vi "DP-Plot I-O.vi"(0 "Input Array (4xn)":dbl[][](array[numeric]) format="%.2f") -> (1 "Current I-O Plot":cluster{cluster{dbl, dbl}[]}[](graph), 2 "All-freq I-O Plot":cluster{cluster{dbl, dbl}[]}[](graph))   [LabVIEW 2020]
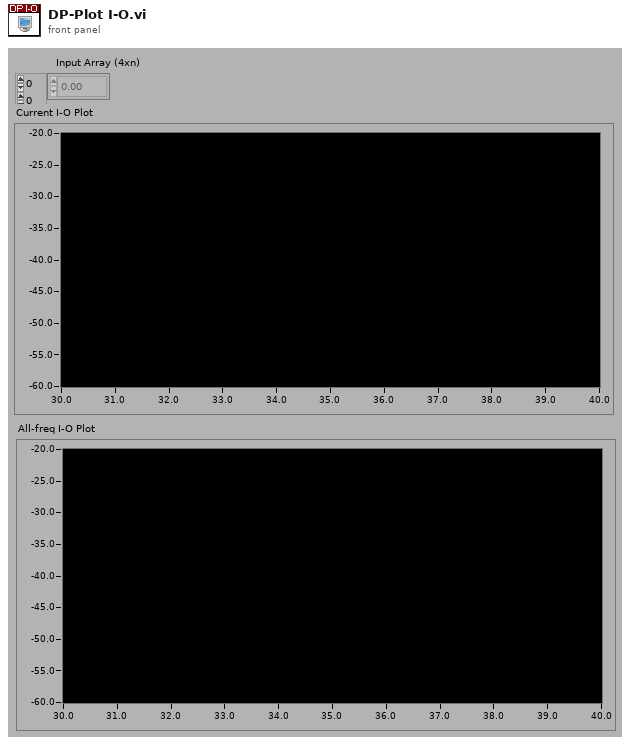
[diagram p1: front panel]
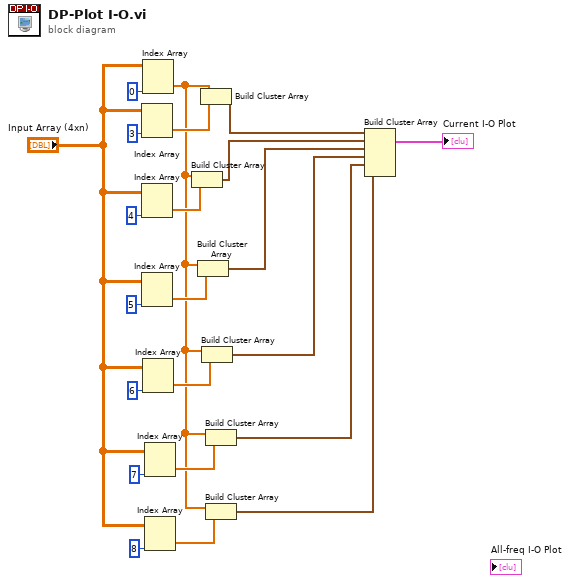
[diagram p0: block diagram]
diagram:
  n1 = Index Array(array="Input Array (4xn)", index (col)=3) -> (element=w20:dbl[])  [unwired: 1 in]
  n2 = Index Array(array="Input Array (4xn)", index (col)=4) -> (element=w21:dbl[])  [unwired: 1 in]
  n3 = Index Array(array="Input Array (4xn)", index (col)=5) -> (element=w14:dbl[])  [unwired: 1 in]
  n4 = Index Array(array="Input Array (4xn)", index (col)=0) -> (element=w2:dbl[])  [unwired: 1 in]
  n5 = Index Array(array="Input Array (4xn)", index (col)=6) -> (element=w12:dbl[])  [unwired: 1 in]
  n6 = Index Array(array="Input Array (4xn)", index (col)=7) -> (element=w7:dbl[])  [unwired: 1 in]
  n7 = Index Array(array="Input Array (4xn)", index (col)=8) -> (element=w5:dbl[])  [unwired: 1 in]
  n8 = Build Cluster Array(w2, w21) -> (w16:cluster{dbl, dbl}[])
  n9 = Build Cluster Array(w2, w14) -> (w13:cluster{dbl, dbl}[])
  n10 = Build Cluster Array(w2, w20) -> (w22:cluster{dbl, dbl}[])
  n11 = Build Cluster Array(w2, w12) -> (w10:cluster{dbl, dbl}[])
  n12 = Build Cluster Array(w2, w7) -> (w6:cluster{dbl, dbl}[])
  n13 = Build Cluster Array(w2, w5) -> (w1:cluster{dbl, dbl}[])
  n14 = Build Cluster Array(w22, w16, w13, w10, w6, w1) -> (→"Current I-O Plot":cluster{cluster{dbl, dbl}[]}[])
